vi "Run_Core.vi"(0 "Booelan Operations in":refnum<class "Boolean Operations.lvclass">, 11 "error in (no error)":errorcluster) -> (4 "Booelan Operations out":refnum<class "Boolean Operations.lvclass">, 6 "Return":variant, 15 "error out":errorcluster)   [LabVIEW 2016, in "Boolean Operations.lvclass"]
uses:
  Boolean Operations.lvclass
  D:/TOOLS/Funtion_Lists/source code/LSL components/functions/functionsbase/functionbase.lvclass
  functionsbase/functionbase.lvclass/functionbase.ctl
  Boolean Operations.lvclass/Boolean Operations.ctl
  functionsbase/properties/Read Smart Syntax Representation.vi
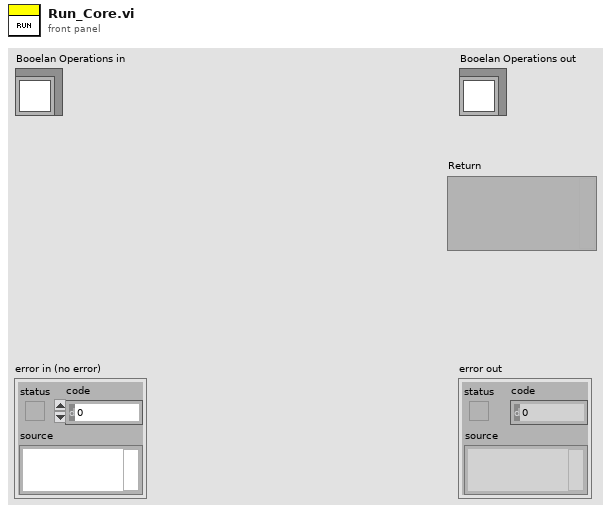
[diagram p1: front panel]
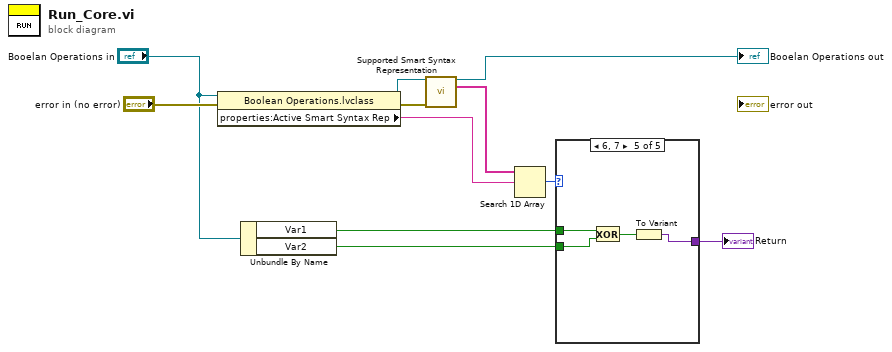
[diagram p0: block diagram]
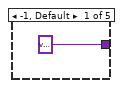
[diagram p2: hidden frame]
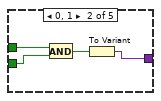
[diagram p3: hidden frame]
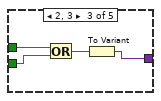
[diagram p4: hidden frame]
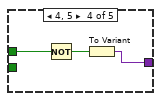
[diagram p5: hidden frame]
diagram:
  n1 = property class="Boolean Operations.lvclass"(reference="Booelan Operations in", error in="error in (no error)") -> (reference out=w7:refnum<class "Boolean Operations.lvclass">, error out=w10:errorcluster, "properties:Active Smart Syntax Rep"=w4:string)
  n2 = Unbundle By Name("Booelan Operations in") -> ("Var1"=w3:bool, "Var2"=w2:bool)
  n3 = call-dynamic "Supported Smart Syntax Representation.vi"("Booelan Operations in"=w7, "error in (no error)"=w10) -> ("Booelan Operations out"=→"Booelan Operations out":refnum<class "Boolean Operations.lvclass">, "Smart Syntax Representation List"=w9:string[])  [unwired: 11 in, 1 out]
  n4 = Search 1D Array(1D array=w9, element=w4) -> (index of element=w8:i32)  [unwired: 1 in]
  n5 = case shown="6, 7" w8 {
    tunnel: w3 -> [_ w16 w20 w23 w27]
    tunnel: w2 -> [_ w15 w19 _ w26]
    tunnel: [variant ("Variant") w13 w17 w21 w24] -> w1
    frame -1, Default {
    }
    frame 0, 1 {
      n6 = And(x=w16, y=w15) -> (x .and. y?=w14:bool)
      n7 = To Variant(anything=w14) -> (Variant=w13:variant)
    }
    frame 2, 3 {
      n8 = Or(x=w20, y=w19) -> (x .or. y?=w18:bool)
      n9 = To Variant(anything=w18) -> (Variant=w17:variant)
    }
    frame 4, 5 {
      n10 = Not(x=w23) -> (.not. x?=w22:bool)
      n11 = To Variant(anything=w22) -> (Variant=w21:variant)
    }
    frame 6, 7 {
      n12 = Exclusive Or(1:w26, 2:w27) -> (0:w25:bool)
      n13 = To Variant(anything=w25) -> (Variant=w24:variant)
    }
  }
  "Return" <- w1
